vi "Test Field.vi"() -> ()   [LabVIEW 2015]
uses:
  Sudoku Library/TypeDef/Sudoku String.ctl
  Sudoku Library/Sudoku Class/Sudoku Class.lvclass
  Sudoku Library/Sudoku Library.lvlib
panel:
  in  "Sudoku String":T1
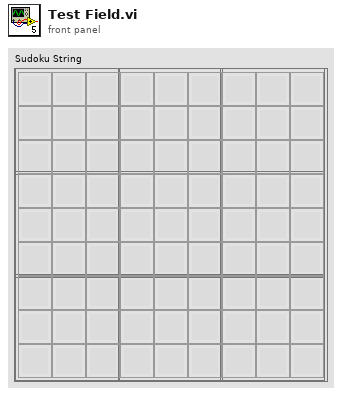
[diagram p1: front panel]
types:
  T1 = typedef "Sudoku Library.lvlib/Sudoku String.ctl" = string[][]
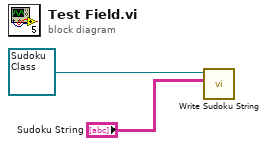
[diagram p0: block diagram]
diagram:
  n1 = call-dynamic "Write Sudoku String.vi"("Sudoku String"="Sudoku String", "Sudoku Class in"=refnum<class "Sudoku Class.lvclass"> refnum ("Sudoku Library:Sudoku Class.lvclass")) -> ()  [unwired: 8 in, 2 out]
